vi "getInterface.vi"(0 "Camera in":refnum<class "Camera.lvclass">, 11 "error in (no error)":errorcluster) -> (4 "Camera out":refnum<class "Camera.lvclass">, 6 "interface":u16(ring)=65535 items=["FireWire"=1, "GenICam"=3, "GigE"=5, "USB"=6, "CameraLinkME4"=7, "USB3"=8, "CLHS"=11, "All"=65535], 15 "error out":errorcluster)   [LabVIEW 2019, in "Camera.lvclass"]
doc: "Gets the interface of the connected camera"
uses:
  Camera.lvclass
  Camera.lvclass/Camera.ctl
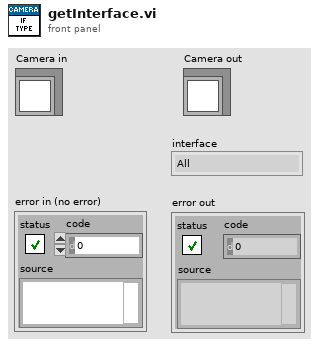
[diagram p1: front panel]
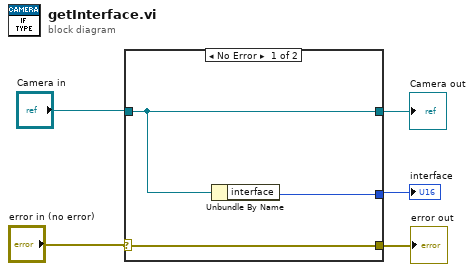
[diagram p0: block diagram]
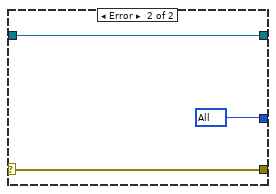
[diagram p2: hidden frame]
diagram:
  n1 = case shown="No Error" "error in (no error)" {
    selector: "error in (no error)" -> [w7 w11]
    tunnel: [w7 w11] -> w3
    tunnel: [w8 w10] -> w4
    tunnel: "Camera in" -> [w8 w10]
    tunnel: [w6 w9] -> w1
    frame No Error {
      n2 = Unbundle By Name(w8) -> ("interface"=w6:u16)
    }
    frame Error {
      w9 = u16 65535 items=["FireWire"=1, "GenICam"=3, "GigE"=5, "USB"=6, "CameraLinkME4"=7, "USB3"=8, "CLHS"=11, "All"=65535] ("interface")
    }
  }
  "error out" <- w3
  "Camera out" <- w4
  "interface" <- w1
